vi "time multiply_v1.vi"() -> ()   [LabVIEW 2020]
uses:
  <vilib>/Analysis/Matrix/Datatypes/RealMatrix.ctl
  <vilib>/Analysis/Matrix/Numeric/Conversions/Array To Matrix - RA.vi
  <vilib>/Analysis/Matrix/Numeric/Conversions/Array To Matrix - RA2.vi
  <vilib>/Analysis/Matrix/Numeric/Multiply/Multiply - RM,RM.vi
  <vilib>/Analysis/Matrix/NI_Matrix.lvlib
panel:
  out "average time":dbl
  out "product":T1
  in  "vector size":i32=20
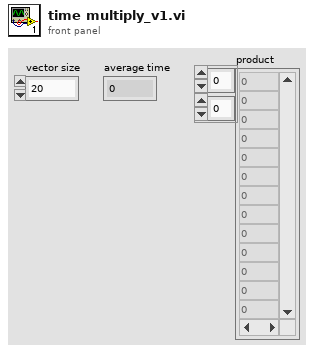
[diagram p1: front panel]
types:
  T1 = typedef "NI_Matrix.lvlib/RealMatrix.ctl" = dbl[][]
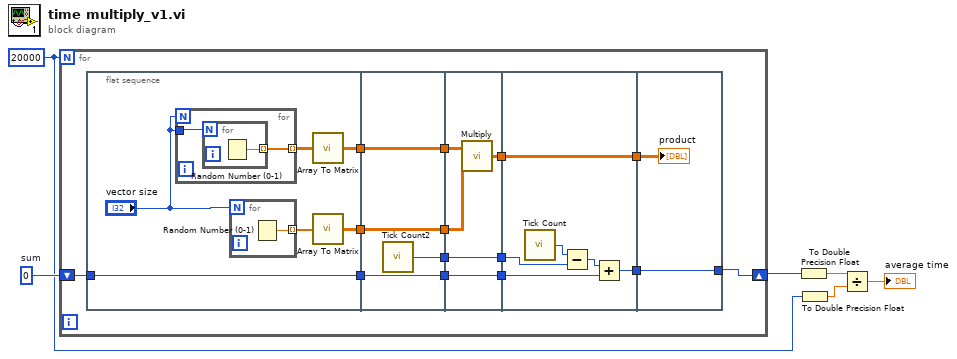
[diagram p0: block diagram]
diagram:
  w6 = u32 0  # sum
  w3 = 20000
  n1 = for {
    N: w3 -> [_]
    shift-right: [w8] -> w5
    shift-left: w6 -> [w9]
    n2 = flat-sequence {
      tunnel: [w25] -> w20
      tunnel: [w23] -> w14
      tunnel: [w21] -> w10
      tunnel: w9 -> [w21]
      tunnel: w20 -> [w34]
      tunnel: [w34] -> w19
      tunnel: [w33] -> w18
      tunnel: [w32] -> w15
      tunnel: w14 -> [w32]
      tunnel: [w31] -> w11
      tunnel: w10 -> [w31]
      tunnel: w19 -> [w37]
      tunnel: w18 -> [w39]
      tunnel: [w39] -> w17
      tunnel: [w36] -> w16
      tunnel: w15 -> [w38]
      tunnel: [w35] -> w12
      tunnel: w11 -> [w35]
      tunnel: w16 -> [w43]
      tunnel: w17 -> [w44]
      tunnel: [w43] -> w13
      tunnel: w12 -> [w41]
      tunnel: [w40] -> w7
      tunnel: w13 -> [w47]
      tunnel: [w46] -> w8
      tunnel: w7 -> [w46]
      frame #0 {
        n3 = for {
          N: "vector size" -> [_]
          tunnel: [w28] -> w24 mode=indexing
          tunnel: "vector size" -> [w27]
          n4 = for {
            N: w27 -> [_]
            tunnel: [w29] -> w28 mode=indexing
            n5 = Random Number (0-1)() -> (number: 0 to 1=w29:dbl)
          }
        }
        n6 = for {
          N: "vector size" -> [_]
          tunnel: [w30] -> w26 mode=indexing
          n7 = Random Number (0-1)() -> (number: 0 to 1=w30:dbl)
        }
        n8 = call-poly <vilib>:"Array To Matrix.vi"("Real 2D Array"=w24) -> ("Real Matrix"=w23:T1)
        n9 = call-poly <vilib>:"Array To Matrix.vi"("Real 1D Array"=w26) -> ("Real Matrix (Column Vector)"=w25:T1)
      }
      frame #1 {
        n10 = call "Tick Count2"() -> ("Tick Count(uSec)"=w33:u32)
      }
      frame #2 {
        n11 = call-poly <vilib>:"Multiply.vi"("Real Matrix B"=w37, "Real Matrix A"=w38) -> ("A * B"=w36:T1)
      }
      frame #3 {
        n12 = call "Tick Count"() -> ("Tick Count(uSec)"=w45:u32)
        n13 = Subtract(x=w45, y=w44) -> (x-y=w42:u32)
        n14 = Add(x=w42, y=w41) -> (x+y=w40:u32)
      }
      frame #4 {
        "product" <- w47
      }
    }
  }
  n15 = To Double Precision Float(number=w5) -> (double precision float=w2:dbl)
  n16 = To Double Precision Float(number=w3) -> (double precision float=w4:dbl)
  n17 = Divide(x=w2, y=w4) -> (x/y=→"average time":dbl)
